vi "Process-ICMP.vi"(9 "Frame":u8[](array[numeric])=[0, 80, 67, 160, 161, 162, 0, 35, 38, 182, 175, 53, 8, 0, 69, 0, 0, 60, 0, 8, 0, 0, 128, 1, 181, 215, 192, 168, 1, 200, 192, 168, 1, 201, 8, 0, 77, 90, 0, 1, 0, 1, 97, 98, 99, 100, 101, 102, 103, 104, 105, 106, 107, 108, 109, 110, 111, 112, 113, 114, 115, 116, 117, 118, 119, 97, 98, 99, 100, 101, 102, 103, 104, 105, 209, 148, 196, 117, 221] format="%02x") -> (1 "Response\nSent":bool)   [LabVIEW 2017]
panel:
  out "Header":T1
  out "ICMP Data":u8[](array[numeric])
  out "Protocol":u8=1
  out "Header\nChecksum Ok?":bool=TRUE
  out "IPv4 Payload":u8[](array[numeric])=[8, 0, 77, 90, 0, 1, 0, 1, 97, 98, 99, 100, 101, 102, 103, 104, 105, 106, 107, 108, 109, 110, 111, 112, 113, 114, 115, 116, 117, 118, 119, 97, 98, 99, 100, 101, 102, 103, 104, 105] format="%02x"
  out "Destination IP":u8[](array[numeric])=[192, 168, 1, 201]
  out "Source IP":u8[](array[numeric])=[192, 168, 1, 200]
  out "Ethernet Payload":u8[](array[numeric])=[69, 0, 0, 60, 0, 8, 0, 0, 128, 1, 181, 215, 192, 168, 1, 200, 192, 168, 1, 201, 8, 0, 77, 90, 0, 1, 0, 1, 97, 98, 99, 100, 101, 102, 103, 104, 105, 106, 107, 108, 109, 110, 111, 112, 113, 114, 115, 116, 117, 118, 119, 97, 98, 99, 100, 101, 102, 103, 104, 105] format="%02x"
  out "Source MAC":u8[](array[numeric])=[0, 35, 38, 182, 175, 53] format="%02x"
  out "Destination MAC":u8[](array[numeric])=[0, 80, 67, 160, 161, 162] format="%02x"
  out "Out Frame":u8[](array[numeric]) format="%02x"
  # "Ethernet II"
  # "IPv4"
  # "ICMP"
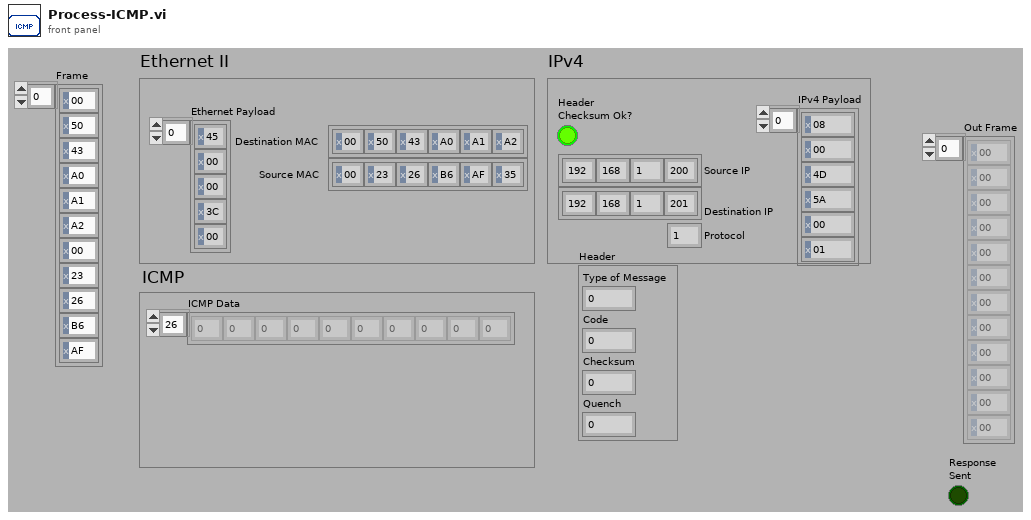
[diagram p1: front panel]
types:
  T1 = cluster{"Type of Message":u8, "Code":u8, "Checksum":u16, "Quench":u32}
  T2 = cluster{"Version":u8, "Header Length":u8, "Total Length":u16, "More Fragments":bool, "Don't Fragment":bool, "Fragment Offset":u16, "TTL":u8, "Header Checksum":u16, "Identification":u16, "Protocol":u8}
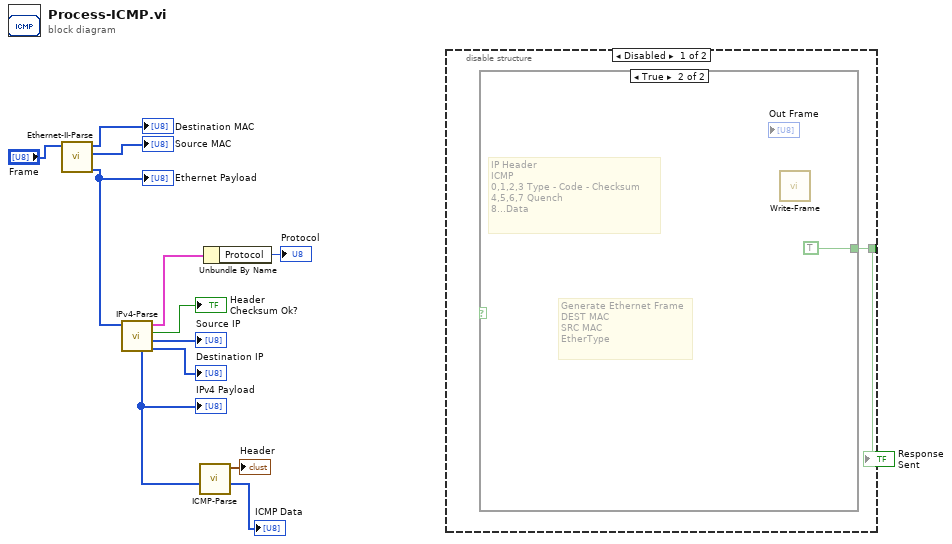
[diagram p0: block diagram]
diagram:
  n1 = call "Ethernet-II-Parse.vi"("Input Frame"="Frame") -> ("Payload"=w7:u8[], "Source MAC"=→"Source MAC":u8[], "Destination MAC"=→"Destination MAC":u8[])  [unwired: 6 in, 2 out]
  "Ethernet Payload" <- w7
  n2 = call "IPv4-Parse.vi"("IPv4 Packet (in)"=w7) -> ("Destination IP"=→"Destination IP":u8[], "Source IP"=→"Source IP":u8[], "Header\nChecksum\nOk?"=→"Header\nChecksum Ok?":bool, "Header"=w5:T2, "IPv4 Payload"=w3:u8[])  [unwired: 6 in]
  "IPv4 Payload" <- w3
  n3 = call "ICMP-Parse.vi"("IPv4 Payload"=w3) -> ("Data"=→"ICMP Data":u8[], "Header"=→"Header":T1)  [unwired: 8 in, 1 out]
  n4 = Unbundle By Name(w5) -> ("Protocol"=→"Protocol":u8)
  n5 = disable-structure shown="Disabled" {
    disable-tunnel: [w14 _] -> w13
    frame Disabled {
      n6 = case shown="True" {
        selector: _ -> [_ _]
        tunnel: [_ TRUE] -> w14
        frame False {
        }
        frame True {
          # "Generate Ethernet Frame\nDEST MAC\nSRC MAC\nEtherType"
          # "IP Header\nICMP\n0,1,2,3 Type - Code - Checksum\n4,5,6,7 Quench\n8...Data"
          n7 = call "Write-Frame.vi"() -> ()  [unwired: 10 in, 2 out]
        }
      }
    }
    frame Enabled {
    }
  }
  "Response\nSent" <- w13
